vi "visualizacionejes - Copy.vi"() -> ()   [LabVIEW 2017]
uses:
  <vilib>/Motion/Express/_s/nimc.fb.read.readExecutionData.axis.vi
  <vilib>/Motion/Express/_s/nimc.fb.arcMove.startArcMove.coordinate.modeCircular.0.vi
  <vilib>/Motion/Express/_s/nimc.fb.straightLineMove.startStraightLineMove.axis.modeAbsolute.0.vi
  <vilib>/Motion/BlockNode/FB.NIMotion.xnode
panel:
  in  "Array":T1(array[cluster])=[{"Motion Resource"="Eje X", "Enum"=enum."lineal", "Array 2"=[0.0, 100.0]}, {"Motion Resource"="Eje Y", "Enum"=enum."lineal", "Array 2"=[80.0, 100.0]}, {"Motion Resource"="Eje X", "Enum"=enum."lineal", "Array 2"=[50.0, 100.0]}, {"Motion Resource"="Eje Y", "Enum"=enum."lineal", "Array 2"=[60.0, 100.0]}, {"Motion Resource"="Eje X", "Enum"=enum."lineal", "Array 2"=[20.0, 100.0]}, {"Motion Resource"="Eje Y", "Enum"=enum."lineal", "Array 2"=[20.0, 100.0]}, {"Motion Resource"="Eje X", "Enum"=enum."lineal", "Array 2"=[40.0, 100.0]}, {"Motion Resource"="Eje Y", "Enum"=enum."lineal", "Array 2"=[-20.0, 100.0]}, {"Motion Resource"="Eje X", "Enum"=enum."lineal", "Array 2"=[20.0, 100.0]}, {"Motion Resource"="Eje Y", "Enum"=enum."lineal", "Array 2"=[-60.0, 100.0]}, {"Motion Resource"="Eje X", "Enum"=enum."lineal", "Array 2"=[49.0, 100.0]}, {"Motion Resource"="Eje Y", "Enum"=enum."lineal", "Array 2"=[-80.0, 100.0]}, {"Motion Resource"="Eje X", "Enum"=enum."lineal", "Array 2"=[0.0, 100.0]}, {"Motion Resource"="Eje Y", "Enum"=enum."lineal", "Array 2"=[0.0, 100.0]}, {"Motion Resource"="Eje Y", "Enum"=enum."lineal", "Array 2"=[-80.0, 100.0]}, {"Motion Resource"="Eje X", "Enum"=enum."lineal", "Array 2"=[70.0, 100.0]}, {"Motion Resource"="Eje Y", "Enum"=enum."lineal", "Array 2"=[80.0, 100.0]}, {"Motion Resource"="Eje X", "Enum"=enum."lineal", "Array 2"=[90.0, 100.0]}, {"Motion Resource"="Coordinate Space 1", "Enum"=enum."Circular", "Array 2"=[40.0, 90.0, -180.0, 100.0]}, {"Motion Resource"="Eje Y", "Enum"=enum."lineal", "Array 2"=[60.0, 100.0]}, {"Motion Resource"="Coordinate Space 1", "Enum"=enum."Circular", "Array 2"=[20.0, 90.0, -180.0, 100.0]}, {"Motion Resource"="Eje Y", "Enum"=enum."lineal", "Array 2"=[0.0, 100.0]}, {"Motion Resource"="Eje X", "Enum"=enum."lineal", "Array 2"=[90.0, 100.0]}, {"Motion Resource"="Coordinate Space 1", "Enum"=enum."Circular", "Array 2"=[100.0, 55.0, -53.7, 100.0]}, {"Motion Resource"="Eje X", "Enum"=enum."lineal", "Array 2"=[110.0, 100.0]}, {"Motion Resource"="Coordinate Space 1", "Enum"=enum."Circular", "Array 2"=[100.0, -53.7, 55.0, 100.0]}, {"Motion Resource"="Eje X", "Enum"=enum."lineal", "Array 2"=[90.0, 100.0]}, {"Motion Resource"="Eje Y", "Enum"=enum."lineal", "Array 2"=[-80.0, 100.0]}, {"Motion Resource"="Eje X", "Enum"=enum."lineal", "Array 2"=[70.0, 100.0]}, {"Motion Resource"="Eje X", "Enum"=enum."lineal", "Array 2"=[150.0, 100.0]}, {"Motion Resource"="Eje Y", "Enum"=enum."lineal", "Array 2"=[80.0, 100.0]}, {"Motion Resource"="Eje X", "Enum"=enum."lineal", "Array 2"=[170.0, 100.0]}, {"Motion Resource"="Eje Y", "Enum"=enum."lineal", "Array 2"=[-80.0, 100.0]}, {"Motion Resource"="Eje X", "Enum"=enum."lineal", "Array 2"=[150.0, 100.0]}, {"Motion Resource"="Eje X", "Enum"=enum."lineal", "Array 2"=[190.0, 100.0]}, {"Motion Resource"="Eje Y", "Enum"=enum."lineal", "Array 2"=[80.0, 100.0]}, {"Motion Resource"="Eje X", "Enum"=enum."lineal", "Array 2"=[210.0, 100.0]}, {"Motion Resource"="Eje Y", "Enum"=enum."lineal", "Array 2"=[20.0, 100.0]}, {"Motion Resource"="Eje X", "Enum"=enum."lineal", "Array 2"=[230.0, 100.0]}, {"Motion Resource"="Eje Y", "Enum"=enum."lineal", "Array 2"=[80.0, 100.0]}, {"Motion Resource"="Eje X", "Enum"=enum."lineal", "Array 2"=[250.0, 100.0]}, {"Motion Resource"="Eje Y", "Enum"=enum."lineal", "Array 2"=[20.0, 100.0]}, {"Motion Resource"="Eje X", "Enum"=enum."lineal", "Array 2"=[230.0, 100.0]}, {"Motion Resource"="Eje Y", "Enum"=enum."lineal", "Array 2"=[0.0, 100.0]}, {"Motion Resource"="Eje X", "Enum"=enum."lineal", "Array 2"=[250.0, 100.0]}, {"Motion Resource"="Eje Y", "Enum"=enum."lineal", "Array 2"=[-80.0, 100.0]}, {"Motion Resource"="Eje X", "Enum"=enum."lineal", "Array 2"=[230.0, 100.0]}, {"Motion Resource"="Eje Y", "Enum"=enum."lineal", "Array 2"=[-20.0, 100.0]}, {"Motion Resource"="Eje X", "Enum"=enum."lineal", "Array 2"=[210.0, 100.0]}, {"Motion Resource"="Eje Y", "Enum"=enum."lineal", "Array 2"=[-80.0, 100.0]}, {"Motion Resource"="Eje X", "Enum"=enum."lineal", "Array 2"=[170.0, 100.0]}, {"Motion Resource"="Eje X", "Enum"=enum."lineal", "Array 2"=[0.0, 100.0]}, {"Motion Resource"="Eje Y", "Enum"=enum."lineal", "Array 2"=[0.0, 100.0]}]
  in  "Stop Button":bool=TRUE
  out "Slide 2":dbl(slide)=110.0 scale=-20.0..280.0
  out "Slide":dbl(slide)=-79.64647107 scale=-100.0..100.0
  out "XY Graph":cluster{dbl[], dbl[]}(graph)
  # "final"
  # "here"
  # "0"
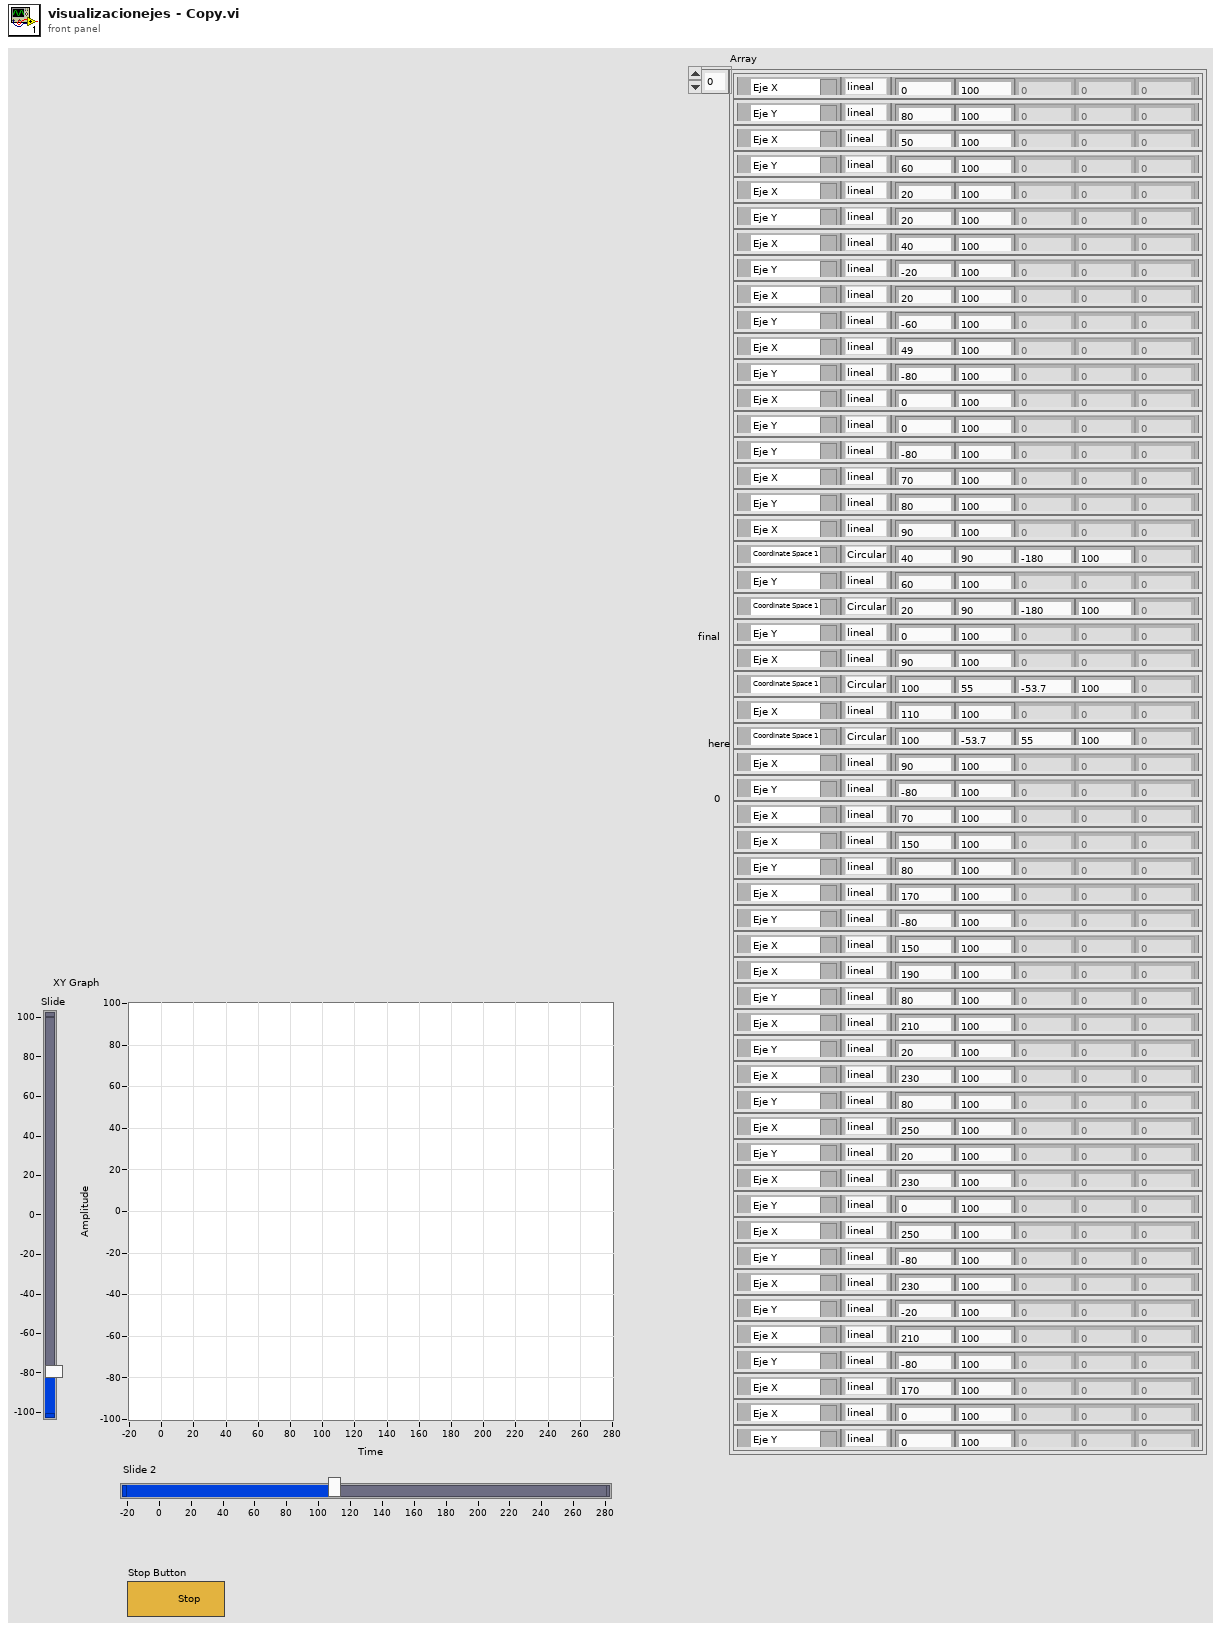
[diagram p1: front panel]
types:
  T1 = cluster{"Motion Resource":refnum<k21>, "Enum":enum16{"Circular", "lineal"}, "Array 2":dbl[]}[]
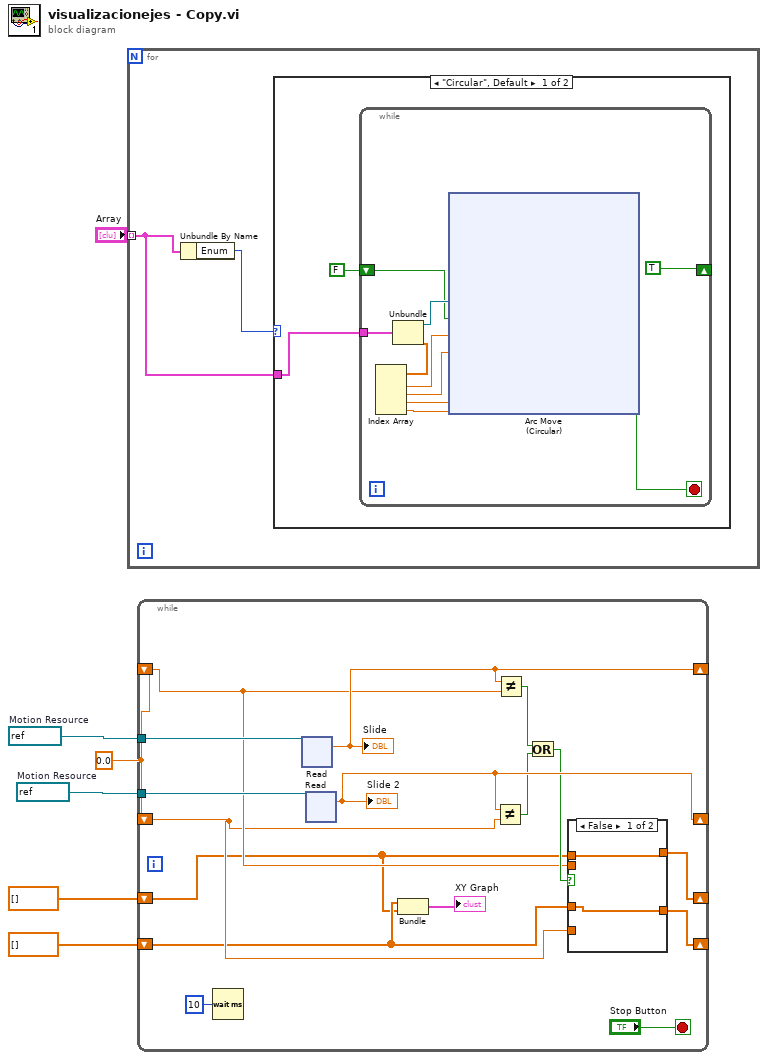
[diagram p0: block diagram]
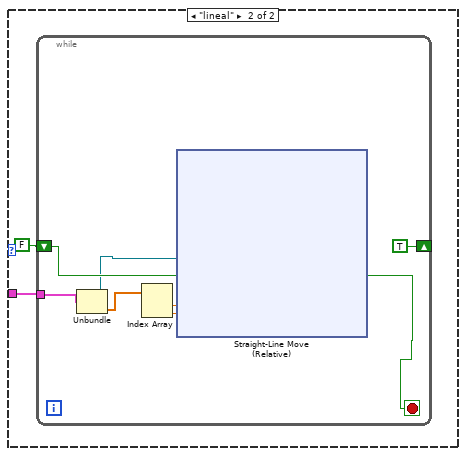
[diagram p2: hidden frame]
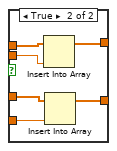
[diagram p3: hidden frame]
diagram:
  w4 = 0.0 ("position")
  w5 = refnum<k21> "Eje X"  # Motion Resource
  w6 = refnum<k21> "Eje Y"  # Motion Resource
  n1 = for {
    tunnel: "Array" -> [w7] mode=indexing
    n2 = Unbundle By Name(w7) -> ("Enum"=w8:enum16{"Circular", "lineal"})
    n3 = case shown="\"Circular\", Default" w8 {
      tunnel: w7 -> [w10 w41]
      frame "Circular", Default {
        n4 = while {
          tunnel: w10 -> [w20]
          shift-right: [TRUE] -> _
          shift-left: FALSE -> [w12]
          stop <- w13 stop-if-true
          n5 = Unbundle(w20) -> ("Motion Resource"=w19:refnum<k21>, "Array 2"=w18:dbl[])  [unwired: 1 out]
          n6 = Index Array(array=w18) -> (element #1=w17:dbl, element #2=w16:dbl, element #3=w15:dbl, element #4=w14:dbl)  [unwired: 4 in]
          n7 = xnode "Arc Move\n(Circular)"("resource"=w19, "execute"=w12, "radius"=w17, "start angle"=w16, "travel angle"=w15, "velocity"=w14) -> ("done"=w13:bool)  [unwired: 2 in, 2 out]
        }
      }
      frame "lineal" {
        n8 = while {
          tunnel: w41 -> [w44]
          shift-right: [TRUE] -> _
          shift-left: FALSE -> [w46]
          stop <- w47 stop-if-true
          n9 = Unbundle(w44) -> ("Motion Resource"=w42:refnum<k21>, "Array 2"=w43:dbl[])  [unwired: 1 out]
          n10 = Index Array(array=w43) -> (element #1=w49:dbl, element #2=w48:dbl)  [unwired: 2 in]
          n11 = xnode "Straight-Line Move\n(Relative)"("resource"=w42, "execute"=w46, "position"=w49, "velocity"=w48) -> ("done"=w47:bool)  [unwired: 2 in, 2 out]
        }
      }
    }
  }
  n12 = while {
    tunnel: w6 -> [w82]
    tunnel: w5 -> [w81]
    shift-right: [w79] -> _
    shift-left: w4 -> [w72]
    shift-right: [w80] -> _
    shift-left: w4 -> [w73]
    shift-right: [w74] -> _
    shift-left: dbl[] [] -> [w69]
    shift-right: [w75] -> _
    shift-left: dbl[] [] -> [w68]
    stop <- "Stop Button" stop-if-true
    n13 = Wait (ms)(milliseconds to wait=u32 10) -> ()  [unwired: 1 out]
    n14 = xnode "Read"("resource"=w82) -> ("position"=w80:dbl)  [unwired: 2 in, 7 out]
    "Slide" <- w80
    n15 = xnode "Read"("resource"=w81) -> ("position"=w79:dbl)  [unwired: 2 in, 7 out]
    "Slide 2" <- w79
    n16 = Bundle(w69, w68) -> (→"XY Graph":cluster{dbl[], dbl[]})  [unwired: 1 in]
    n17 = Not Equal?(x=w79, y=w72) -> (x != y?=w78:bool)
    n18 = Not Equal?(x=w80, y=w73) -> (x != y?=w77:bool)
    n19 = Or(x=w77, y=w78) -> (x .or. y?=w76:bool)
    n20 = case shown="False" w76 {
      tunnel: w68 -> [w84 w90]
      tunnel: [w84 w89] -> w75
      tunnel: w69 -> [w83 w88]
      tunnel: [w83 w87] -> w74
      tunnel: w73 -> [_ w86]
      tunnel: w72 -> [_ w85]
      frame False {
      }
      frame True {
        n21 = Insert Into Array(array=w90, new element=w86) -> (w89:dbl[])  [unwired: 1 in]
        n22 = Insert Into Array(array=w88, new element=w85) -> (w87:dbl[])  [unwired: 1 in]
      }
    }
  }
